vi "EXO2 Com.vi"() -> ()   [LabVIEW 2016, in "EXO2.lvlib"]
uses:
  EXO2.lvlib
  <vilib>/Instr/_visa.llb/VISA Configure Serial Port (Instr).vi
  <vilib>/regexp/Match Regular Expression.xnode
panel:
  out "EXO message":T1
  in  "stop":bool
  in  "start":bool
  in  "open":bool
  in  "停止":bool
  out "字符串":string
  out "匹配字段":string
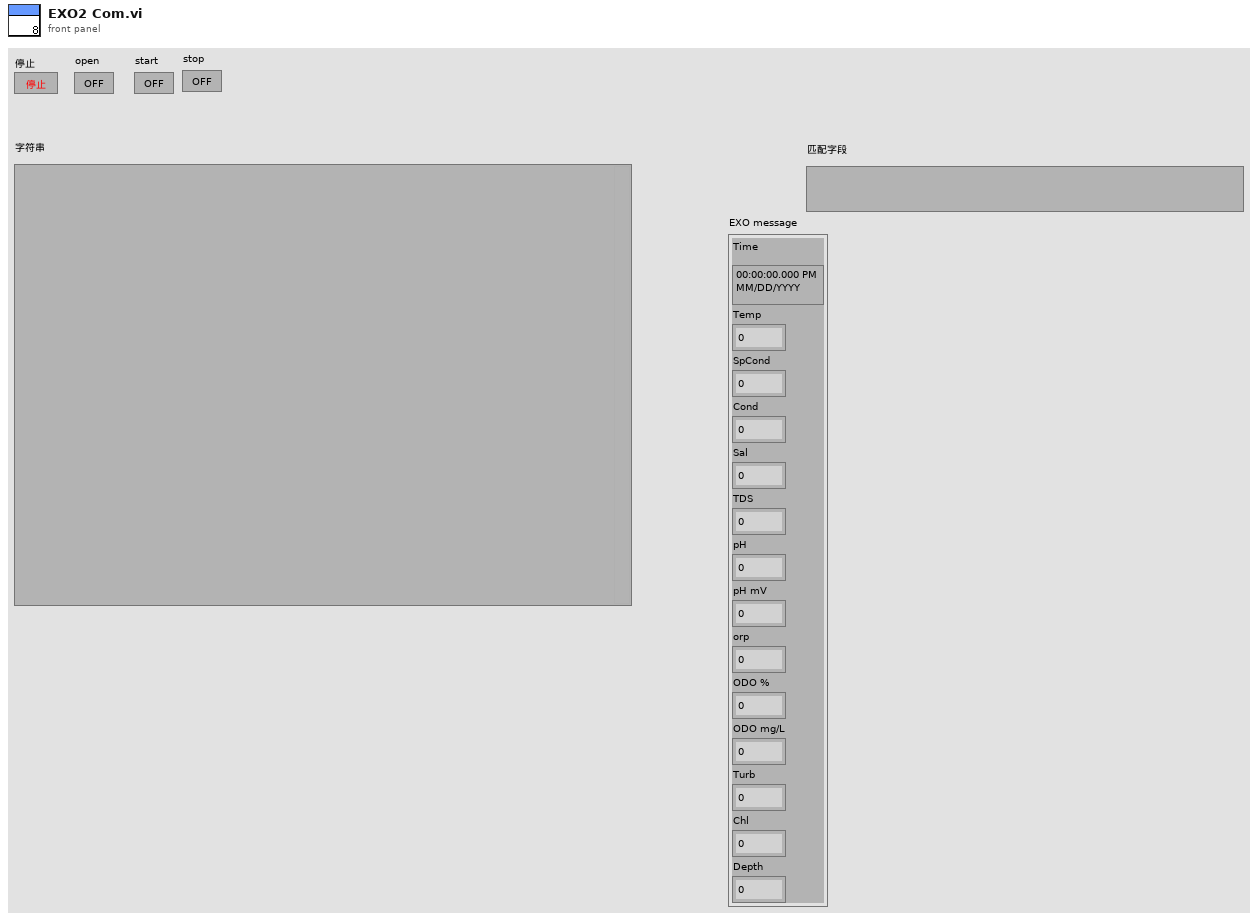
[diagram p1: front panel]
types:
  T1 = cluster{"Time":timestamp, "Temp":dbl, "SpCond":dbl, "Cond":dbl, "Sal":dbl, "TDS":dbl, "pH":dbl, "pH mV":dbl, "orp":dbl, "ODO %":dbl, "ODO mg/L":dbl, "Turb":dbl, "Chl":dbl, "Depth":dbl}
  T2 = enum16{"open", "poll", "close", "run", "stop", "shutdown"}
  T3 = cluster{"Time":timestamp, "Temp":dbl, "SpCond":dbl, "Cond":dbl, "Sal":dbl, "TDS":dbl, "pH":dbl, "pH mV":dbl, "orp":dbl, "ODO %":dbl, "ODO mg/L":dbl, "Turb":dbl, "Chl":dbl, "Depth":dbl}[]
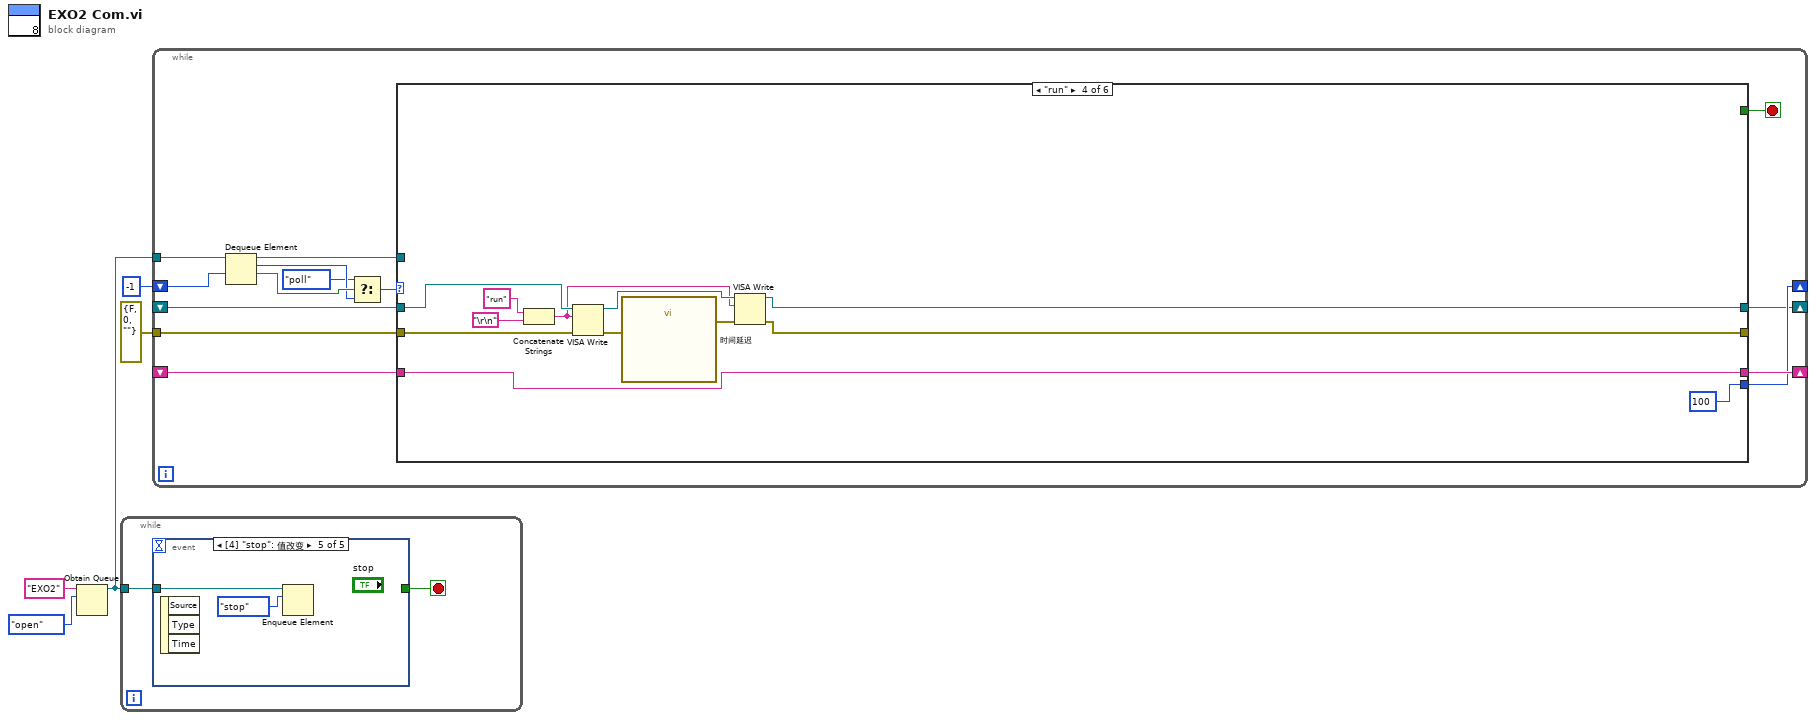
[diagram p0: block diagram]
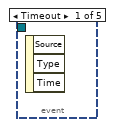
[diagram p2: hidden frame]
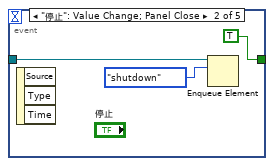
[diagram p3: hidden frame]
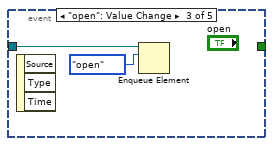
[diagram p4: hidden frame]
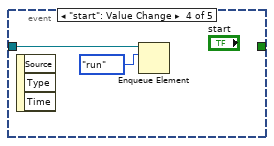
[diagram p5: hidden frame]
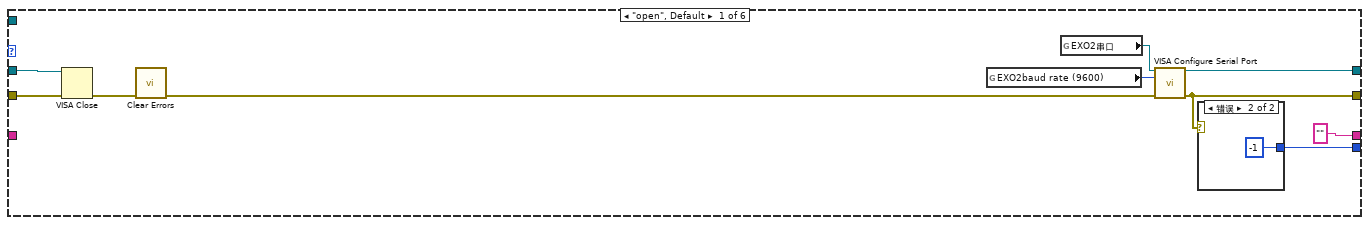
[diagram p6: hidden frame]
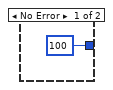
[diagram p7: hidden frame]
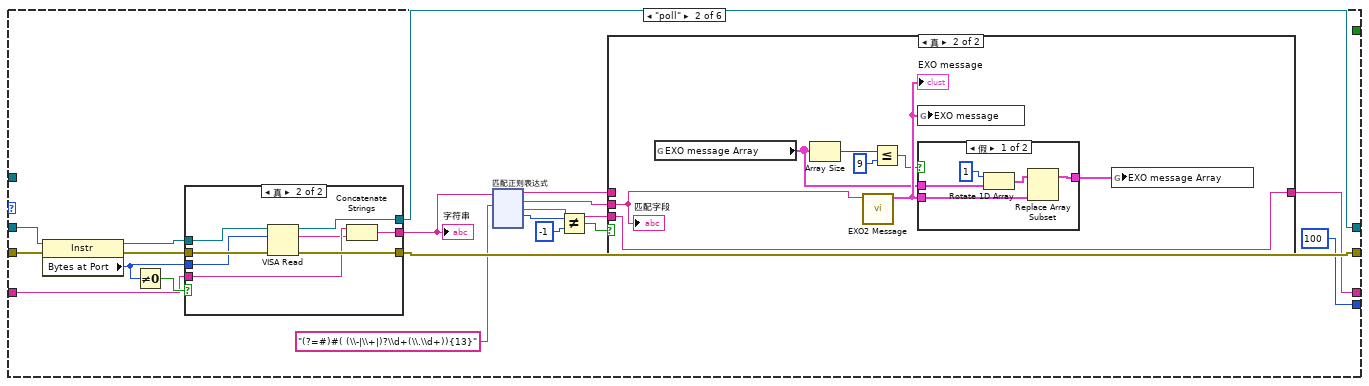
[diagram p8: hidden frame]
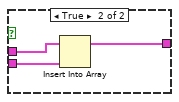
[diagram p10: hidden frame]
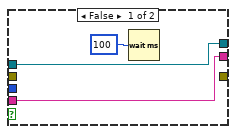
[diagram p11: hidden frame]
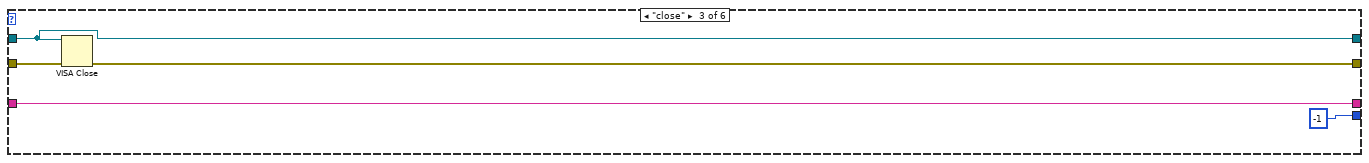
[diagram p12: hidden frame]
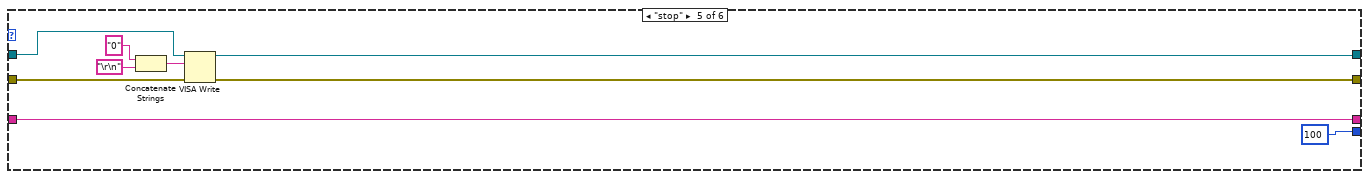
[diagram p13: hidden frame]
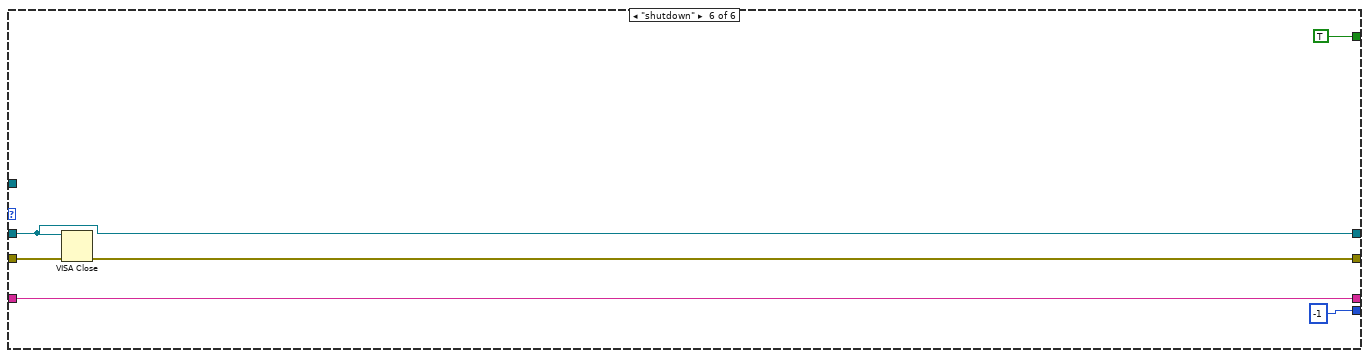
[diagram p14: hidden frame]
diagram:
  n1 = Obtain Queue(name (unnamed)="EXO2" ("名称（未命名）"), element data type=T2."open" ("枚举")) -> (queue out=w3:refnum<queue>)  [unwired: 3 in, 2 out]
  n2 = while {
    tunnel: w3 -> [w6]
    stop <- w7 stop-if-true
    n3 = event shown="[4] \"stop\": 值改变" {
      selector: _ -> [_ _ _ _ _]
      dyn-events: _ -> [_ _ _ _ _]
      timeout: _ -> [_ _ _ _ _]
      tunnel: [_ TRUE _ _ _] -> w7
      tunnel: w6 -> [_ w9 w12 w14 w16]
      event Timeout {
        n4 = event-data() -> ()  [unwired: 1 in, 3 out]
      }
      event "停止": Value Change; Panel Close {
        n5 = event-data() -> ()  [unwired: 1 in, 3 out]
        n6 = Enqueue Element(queue=w9, element=T2."shutdown" ("元素")) -> ()  [unwired: 2 in, 3 out]
      }
      event "open": Value Change {
        n7 = event-data() -> ()  [unwired: 1 in, 3 out]
        n8 = Enqueue Element(queue=w12, element=T2."open" ("元素")) -> ()  [unwired: 2 in, 3 out]
      }
      event "start": Value Change {
        n9 = event-data() -> ()  [unwired: 1 in, 3 out]
        n10 = Enqueue Element(queue=w14, element=T2."run" ("元素")) -> ()  [unwired: 2 in, 3 out]
      }
      event "stop": Value Change {
        n11 = event-data() -> ()  [unwired: 1 in, 3 out]
        n12 = Enqueue Element(queue=w16, element=T2."stop" ("元素")) -> ()  [unwired: 2 in, 3 out]
      }
    }
  }
  n13 = while {
    tunnel: w3 -> [w30]
    shift-right: [w17] -> _
    shift-left: _ -> [w28]
    shift-right: [w27] -> _
    shift-left: _ -> [w26]
    tunnel: errorcluster {"status"=FALSE, "code"=0, "source"=""} ("错误输入（无错误）") -> [w24]
    shift-right: [w22] -> _
    shift-left: -1 ("超时毫秒(-1)") -> [w23]
    stop <- w25 stop-if-true
    n14 = Dequeue Element(queue=w30, timeout in ms (-1)=w23) -> (queue out=w29:refnum<queue>, element=w20:T2, timed out?=w21:bool)  [unwired: 1 in, 1 out]
    n15 = Select(t=T2."poll", s=w21, f=w20) -> (s? t:f=w19:T2)
    n16 = case shown="\"run\"" w19 {
      tunnel: w29 -> [_ _ _ _ _ _]
      tunnel: [w40 w56 w208 w211 w225 w235] -> w17
      tunnel: w28 -> [w39 w57 w208 w218 w227 w235]
      tunnel: ["" ("String") w44 w207 w220 w229 w233] -> w27
      tunnel: w26 -> [_ w55 w207 w220 w229 w233]
      tunnel: [_ _ _ _ _ TRUE] -> w25
      tunnel: w24 -> [w37 w53 w206 w217 w226 w232]
      tunnel: [w36 w54 w205 w210 w224 w231] -> _
      tunnel: [w35 100 ("超时毫秒(-1)") -1 ("超时毫秒(-1)") 100 ("超时毫秒(-1)") 100 ("超时毫秒(-1)") -1 ("超时毫秒(-1)")] -> w22
      frame "open", Default {
        n17 = VISA Close(VISA resource name=w39, error in (no error)=w37) -> (error out=w34:errorcluster)
        n18 = call <vilib>:"Clear Errors.vi"("error in (no error)"=w34) -> ("error out"=w33:errorcluster)  [unwired: 5 in, 1 out]
        n19 = global read "EXO2全局变量.vi" "EXO2baud rate (9600)"() -> (w32:u32)
        n20 = global read "EXO2全局变量.vi" "EXO2串口"() -> (w31:refnum<visa-resource-name>)
        n21 = call-poly "VISA Configure Serial Port"("VISA resource name"=w31, "baud rate (9600)"=w32, "error in (no error)"=w33) -> ("VISA resource name out"=w40:refnum<visa-resource-name>, "error out"=w36:errorcluster)  [unwired: 11 in]
        n22 = case shown="错误" w36 {
          tunnel: [100 ("超时毫秒(-1)") -1 ("超时毫秒(-1)")] -> w35
          frame No Error {
          }
          frame Error {
          }
        }
      }
      frame "poll" {
        n23 = property class="Instr"(reference=w57, error in=w53) -> (reference out=w59:refnum<visa-resource-name>, error out=w60:errorcluster, "Bytes at Port"=w61:u32)
        n24 = Not Equal To 0?(x=w61) -> (x != 0?=w58:bool)
        n25 = case shown="真" w58 {
          tunnel: w59 -> [w195 w203]
          tunnel: w60 -> [_ w202]
          tunnel: [w195 w201] -> w56
          tunnel: [_ w200] -> w54
          tunnel: [w193 w197] -> w50
          tunnel: w55 -> [w193 w199]
          tunnel: w61 -> [_ w196]
          frame False {
            n26 = Wait (ms)(milliseconds to wait=u32 100 ("等待时间（毫秒）")) -> ()  [unwired: 1 out]
          }
          frame True {
            n27 = VISA Read(VISA resource name=w203, byte count=w196, error in (no error)=w202) -> (VISA resource name out=w201:refnum<visa-resource-name>, read buffer=w198:string, error out=w200:errorcluster)  [unwired: 1 out]
            n28 = Concatenate Strings(w199, w198) -> (w197:string)
          }
        }
        "字符串" <- w50
        n29 = xnode "匹配正则表达式"("输入字符串"=w50, "正则表达式"="(?=#)#( (\\-|\\+|)?\\d+(\\.\\d+)){13}") -> ("匹配之前"=w43:string, "所有匹配"=w46:string, "匹配之后"=w45:string, "匹配后偏移量"=w49:i32)  [unwired: 4 in, 1 out]
        n30 = Not Equal?(x=w49, y=-1) -> (x != y?=w47:bool)
        n31 = case shown="真" w47 {
          tunnel: [w176 w184] -> w44
          tunnel: w46 -> [_ w183]
          tunnel: w45 -> [_ w184]
          tunnel: w43 -> [w176 _]
          frame False {
          }
          frame True {
            n32 = global read "EXO2全局变量.vi" "EXO message Array"() -> (w180:T3)
            n33 = Array Size(array=w180) -> (size(s)=w179:i32)
            n34 = call "EXO2 Message.vi"("字符串"=w183) -> ("EXO message"=w182:T1)  [unwired: 9 in, 1 out]
            "EXO message" <- w182
            n35 = Less Or Equal?(x=w179, y=9) -> (x <= y?=w177:bool)
            n36 = global write "EXO2全局变量.vi" "EXO message"(w182) -> ()
            n37 = case shown="假" w177 {
              tunnel: w182 -> [w186 w192]
              tunnel: [w185 w191] -> w181
              tunnel: w180 -> [w189 w190]
              frame False {
                n38 = Rotate 1D Array(1:w189, 2:1 ("n")) -> (0:w187:T3)
                n39 = Replace Array Subset(array=w187, new element=w186) -> (w185:T3)  [unwired: 1 in]
              }
              frame True {
                n40 = Insert Into Array(array=w190, new element=w192) -> (w191:T3)  [unwired: 1 in]
              }
            }
            n41 = global write "EXO2全局变量.vi" "EXO message Array"(w181) -> ()
            "匹配字段" <- w183
          }
        }
      }
      frame "close" {
        n42 = VISA Close(VISA resource name=w208, error in (no error)=w206) -> (error out=w205:errorcluster)
      }
      frame "run" {
        n43 = Concatenate Strings("run" ("写入缓冲区"), "\r\n") -> (w209:string)
        n44 = VISA Write(VISA resource name=w218, write buffer=w209, error in (no error)=w217) -> (VISA resource name out=w212:refnum<visa-resource-name>, error out=w214:errorcluster)  [unwired: 1 out]
        n45 = call "时间延迟"("error in (no error)"=w214) -> ("error out"=w213:errorcluster)  [unwired: 10 in]
        n46 = VISA Write(VISA resource name=w212, write buffer=w209, error in (no error)=w213) -> (VISA resource name out=w211:refnum<visa-resource-name>, error out=w210:errorcluster)  [unwired: 1 out]
      }
      frame "stop" {
        n47 = Concatenate Strings("0" ("写入缓冲区"), "\r\n") -> (w221:string)
        n48 = VISA Write(VISA resource name=w227, write buffer=w221, error in (no error)=w226) -> (VISA resource name out=w225:refnum<visa-resource-name>, error out=w224:errorcluster)  [unwired: 1 out]
      }
      frame "shutdown" {
        n49 = VISA Close(VISA resource name=w235, error in (no error)=w232) -> (error out=w231:errorcluster)
      }
    }
  }
